vi "AvoidObstacle.vi"() -> (2 "Output Movement (Test Later)":T1(ring), 3 "Output Speed":dbl)   [LabVIEW 2017]
uses:
  IR_global.vi
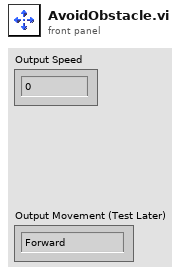
[diagram p1: front panel]
types:
  T1 = enum16{"Forward", "Backward", "Left", "Right", "Rotate Left", "Rotate Right"}
  T2 = enum16{"Forward", "Backward", "Left", "Right", "Rotate Left", "Rotate Right"}[]
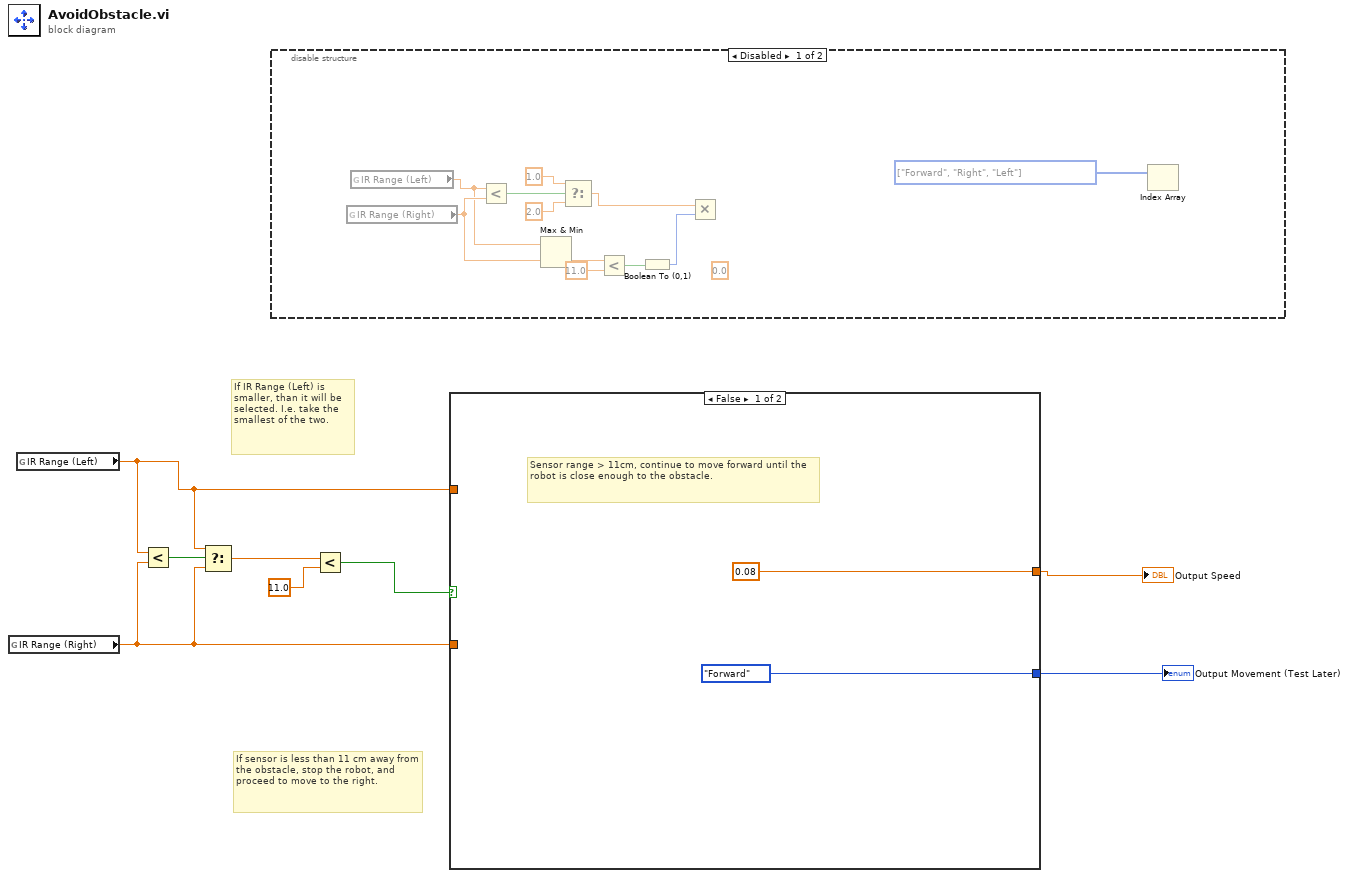
[diagram p0: block diagram]
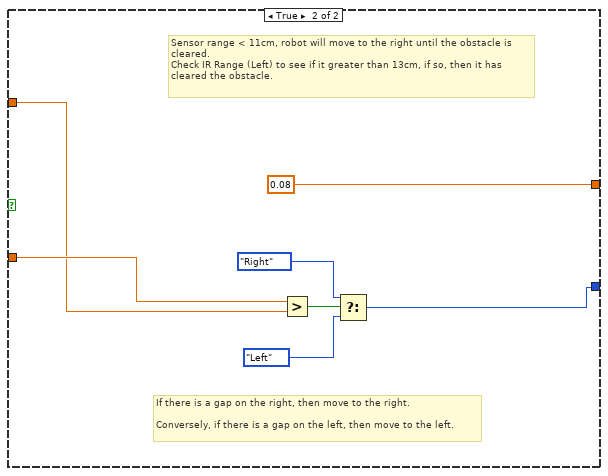
[diagram p2: hidden frame]
diagram:
  # "If sensor is less than 11 cm away from the obstacle, stop the robot, and proceed to move to the right."
  # "If IR Range (Left) is smaller, than it will be selected. I.e. take the smallest of the two."
  n1 = global read "IR_global.vi" "IR Range (Right)"() -> (w3:dbl)
  n2 = global read "IR_global.vi" "IR Range (Left)"() -> (w2:dbl)
  n3 = Less?(x=w2, y=w3) -> (x < y?=w8:bool)
  n4 = Select(t=w2, s=w8, f=w3) -> (s? t:f=w7:dbl)
  n5 = disable-structure shown="Disabled" {
    frame Disabled {
      (unwired) 0.0 ("Output Speed")
      w19 = T2 [enum."Forward", enum."Right", enum."Left"] items=["Forward", "Backward", "Left", "Right", "Rotate Left", "Rotate Right"]
      n6 = global read "IR_global.vi" "IR Range (Right)"() -> (w15:dbl)
      n7 = global read "IR_global.vi" "IR Range (Left)"() -> (w14:dbl)
      n8 = Less?(x=w14, y=w15) -> (x < y?=w18:bool)
      n9 = Max & Min(x=w14, y=w15) -> (min(x,y)=w13:dbl)  [unwired: 1 out]
      n10 = Select(t=1.0, s=w18, f=2.0) -> (s? t:f=w10:dbl)
      n11 = Less?(x=w13, y=11.0) -> (x < y?=w11:bool)
      n12 = Boolean To (0,1)(Boolean=w11) -> (0, 1=w9:i16)
      n13 = Multiply(x=w10, y=w9) -> ()  [unwired: 1 out]
      n14 = Index Array(array=w19) -> ()  [unwired: 1 in, 1 out]
    }
    frame Enabled {
    }
  }
  n15 = Less?(x=w7, y=11.0) -> (x < y?=w5:bool)
  n16 = case shown="False" w5 {
    tunnel: [T1."Forward" ("Output Movement") w22] -> w4
    tunnel: [0.08 ("Output Speed") 0.08 ("Output Speed")] -> w1
    tunnel: w3 -> [_ w27]
    tunnel: w2 -> [_ w26]
    frame False {
      # "Sensor range > 11cm, continue to move forward until the robot is close enough to the obstacle."
    }
    frame True {
      # "If there is a gap on the right, then move to the right.\n\nConversely, if there is a gap on the left, then move to the left."
      # "Sensor range < 11cm, robot will move to the right until the obstacle is cleared.\nCheck IR Range (Left) to see if it greater than 13cm, if so, then it has cleared the obstacle."
      n17 = Greater?(x=w27, y=w26) -> (0:w25:bool)
      n18 = Select(t=T1."Right" ("Output Movement"), s=w25, f=T1."Left" ("Output Movement")) -> (s? t:f=w22:T1)
    }
  }
  "Output Movement (Test Later)" <- w4
  "Output Speed" <- w1
